vi "Waveforms.vi"(7 "amplitude 4":dbl=1.0 format="%0.2p", 8 "Error In":errorcluster, 9 "amplitude 3":dbl=1.0 format="%0.2p", 10 "amplitude 2":dbl=1.0 format="%0.2p", 11 "amplitude 1":dbl=1.0 format="%0.2p") -> (0 "Error Out":errorcluster, 1 "signal 3":waveform(dbl), 2 "signal 2":waveform(dbl), 3 "signal 1":waveform(dbl), 5 "signal 4":waveform(dbl))   [LabVIEW 2023, in "Waveforms.lvlib"]
doc: "Demonstrates how to use the LabVIEW Unit Test Framework Toolkit to check VIs which contain arrays or clusters for functional correctness. The test file for this VI, Waveforms.lvtest, is configured to fail."
uses:
  Waveforms.lvlib
  <vilib>/measure/NI_MABase.lvlib
panel:
  # "Overview: Demonstrates how to use the LabVIEW Unit Test Framework Toolkit to check VIs which contain arrays or clusters for functional correctness. \nRequirements: LabVIEW Full Development System, Unit Test Framework Toolkit\nInstructions:\n1.  Execute the Waveforms.lvtest test file for this VI. In the Project Explorer window, expand the Unit Test Files folder, right-click Waveforms.lvtest, and select Run from the shortcut menu.\n2.  View the test results in the Unit Test Framework Results window, which shows that this test fails."
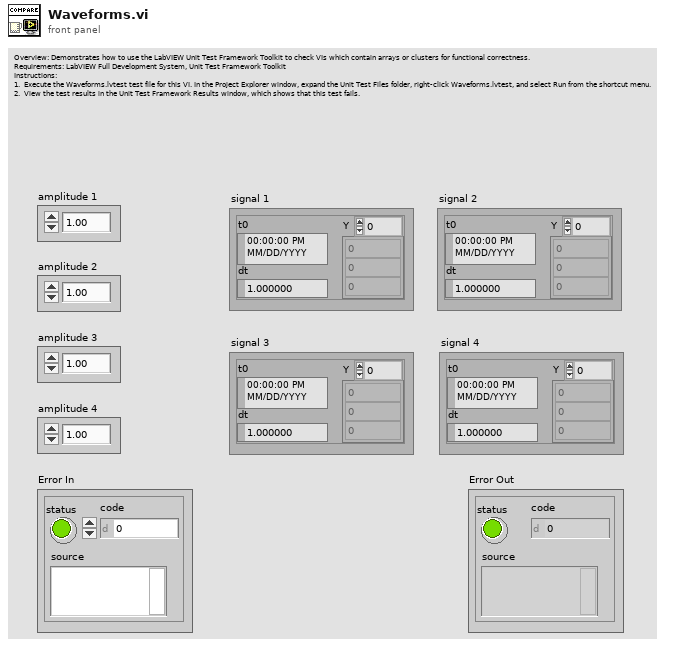
[diagram p1: front panel]
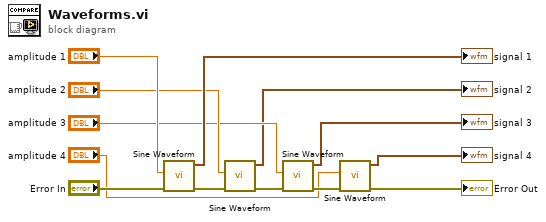
[diagram p0: block diagram]
diagram:
  n1 = call <vilib>:"Sine Waveform.vi"("error in (no error)"="Error In", "amplitude"="amplitude 1") -> ("error out"=w11:errorcluster, "signal out"=→"signal 1":waveform(dbl))  [unwired: 5 in, 3 out]
  n2 = call <vilib>:"Sine Waveform.vi"("error in (no error)"=w11, "amplitude"="amplitude 2") -> ("error out"=w10:errorcluster, "signal out"=→"signal 2":waveform(dbl))  [unwired: 5 in, 3 out]
  n3 = call <vilib>:"Sine Waveform.vi"("error in (no error)"=w10, "amplitude"="amplitude 3") -> ("error out"=w9:errorcluster, "signal out"=→"signal 3":waveform(dbl))  [unwired: 5 in, 3 out]
  n4 = call <vilib>:"Sine Waveform.vi"("error in (no error)"=w9, "amplitude"="amplitude 4") -> ("error out"=→"Error Out":errorcluster, "signal out"=→"signal 4":waveform(dbl))  [unwired: 5 in, 3 out]
